vi "enableComponent.vi"(8 "Error In":errorcluster, 9 "enable":bool, 10 "component":T1=1 items=["Backbone"=1, "Ticks"=2, "Labels"=4], 11 "QwtAbstractScaleDraw In":refnum<class "QwtAbstractScaleDraw.lvclass">) -> (0 "Error Out":errorcluster, 3 "QwtAbstractScaleDraw Out":refnum<class "QwtAbstractScaleDraw.lvclass">)   [LabVIEW 2014, in "QwtAbstractScaleDraw.lvclass"]
doc: "LabVIEW-specific documentation is not yet available. See <b>https://qwt.sourceforge.io/class_qwt_abstract_scale_draw.html#enableComponent</b>"
uses:
  QwtAbstractScaleDraw.lvclass
  ScaleComponent.ctl
  LQ Core/LQIdentity/LQIdentity.lvclass/LQIdentity.ctl
  LQ Core/LQ Core.lvlib
  LQ Core/LQIdentity/LQIdentity.lvclass
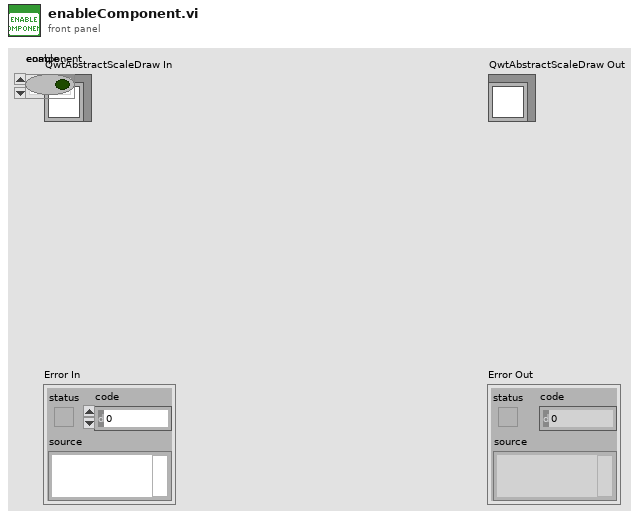
[diagram p1: front panel]
types:
  T1 = typedef "QwtAbstractScaleDraw.lvclass/ScaleComponent.ctl" = i32
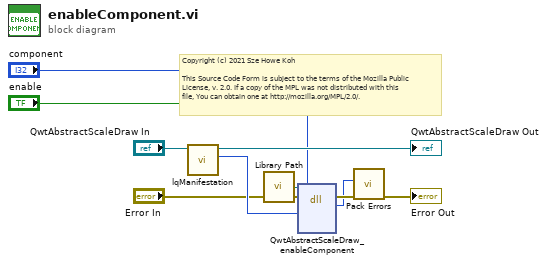
[diagram p0: block diagram]
diagram:
  # "Copyright (c) 2021 Sze Howe Koh\n\nThis Source Code Form is subject to the terms of the Mozilla Public\nLicense, v. 2.0. If a copy of the MPL was not distributed with this\nfile, You can obtain one at http://mozilla.org/MPL/2.0/."
  n1 = call "lqManifestation.vi"("LQIdentity in"="QwtAbstractScaleDraw In") -> ("Manifestation"=w7:u64, "LQIdentity out"=→"QwtAbstractScaleDraw Out":refnum<class "QwtAbstractScaleDraw.lvclass">)  [unwired: 9 in]
  n2 = call "Library Path.vi"() -> ("Library Path"=w8:path)
  n3 = dll-call lib="?" fn="QwtAbstractScaleDraw_enableComponent"(path in=w8, error in="Error In", "_instance"=w7, "component"="component", "enable"="enable") -> (error out=w5:errorcluster, w3:i32)  [unwired: 4 in, 1 out]
  n4 = call "Pack Errors.vi"("Error In"=w5, "Error Code"=w3) -> ("Error Out"=→"Error Out":errorcluster)  [unwired: 9 in]
